vi "Autonomous Independent.vi"   [LabVIEW 2016]
doc: "This VI is called when autonomous begins, and will automatically be terminated when autonomous ends. You can carry out timed or sensor driven robot movement independently without needing to return to the caller."
uses:
  <vilib>/Rock Robotics/WPI/Utilities/WPI_GetSetVariantRefNum.vi
  <vilib>/Rock Robotics/Network Tables/NT Read String.vi
  <vilib>/Rock Robotics/WPI/RobotDrive/WPI_RobotDriveArcadeDrive_Standard(NoSaturation).vi
  <vilib>/Rock Robotics/Network Tables/NT Write Numeric Array.vi
  <vilib>/Rock Robotics/Network Tables/NT Write Boolean.vi
panel:
  # "Be sure to right-click and choose Data Operations>>Make Current Value default if you want to save the array values with the VI"
types:
  T1 = typedef "WPI_JoystickDevRef.ctl" = cluster{"Device":T2}
  T2 = typedef "WPI_JoystickDeviceEnum.ctl" = enum16{"USB 0", "USB 1", "USB 2", "USB 3", "USB 4", "USB 5"}
  T3 = typedef "WPI_RobotDriveDevRef.ctl" = cluster{"DevStatus":errorcluster, "Motors[]":T4[], "Square Inputs":bool, "Max Output":dbl}
  T4 = typedef "WPI_MotorControlDeviceRef.ctl" = cluster{"DeviceStatus":errorcluster, "Type":T5, "PWM":cluster{"PWM Channel":T6, "DeadBand":T7}, "CAN":cluster{"Device Number":u8, "SetOutput VI Ref":variant, "GetOutput VI Ref":variant, "Enable VI Ref":variant, "Disable VI Ref":variant, "Data":variant}, "Invert":bool}
  T5 = typedef "WPI_MotorControlType.ctl" = enum16{"PWM", "CAN"}
  T6 = typedef "FPGA_DIOPWMChannel.ctl" = enum8{"PWM 0", "PWM 1", "PWM 2", "PWM 3", "PWM 4", "PWM 5", "PWM 6", "PWM 7", "PWM 8", "PWM 9", "PWM MXP 0", "PWM MXP 1", "PWM MXP 2", "PWM MXP 3", "PWM MXP 4", "PWM MXP 5", "PWM MXP 6", "PWM MXP 7", "PWM MXP 8", "PWM MXP 9", "Invalid"}
  T7 = typedef "WPI_PWMDeadband.ctl" = cluster{"Name":string, "maxPositivePwm":i32, "minPositivePwm":i32, "centerPwm":i32, "maxNegativePwm":i32, "minNegativePwm":i32, "angularRange":u16}
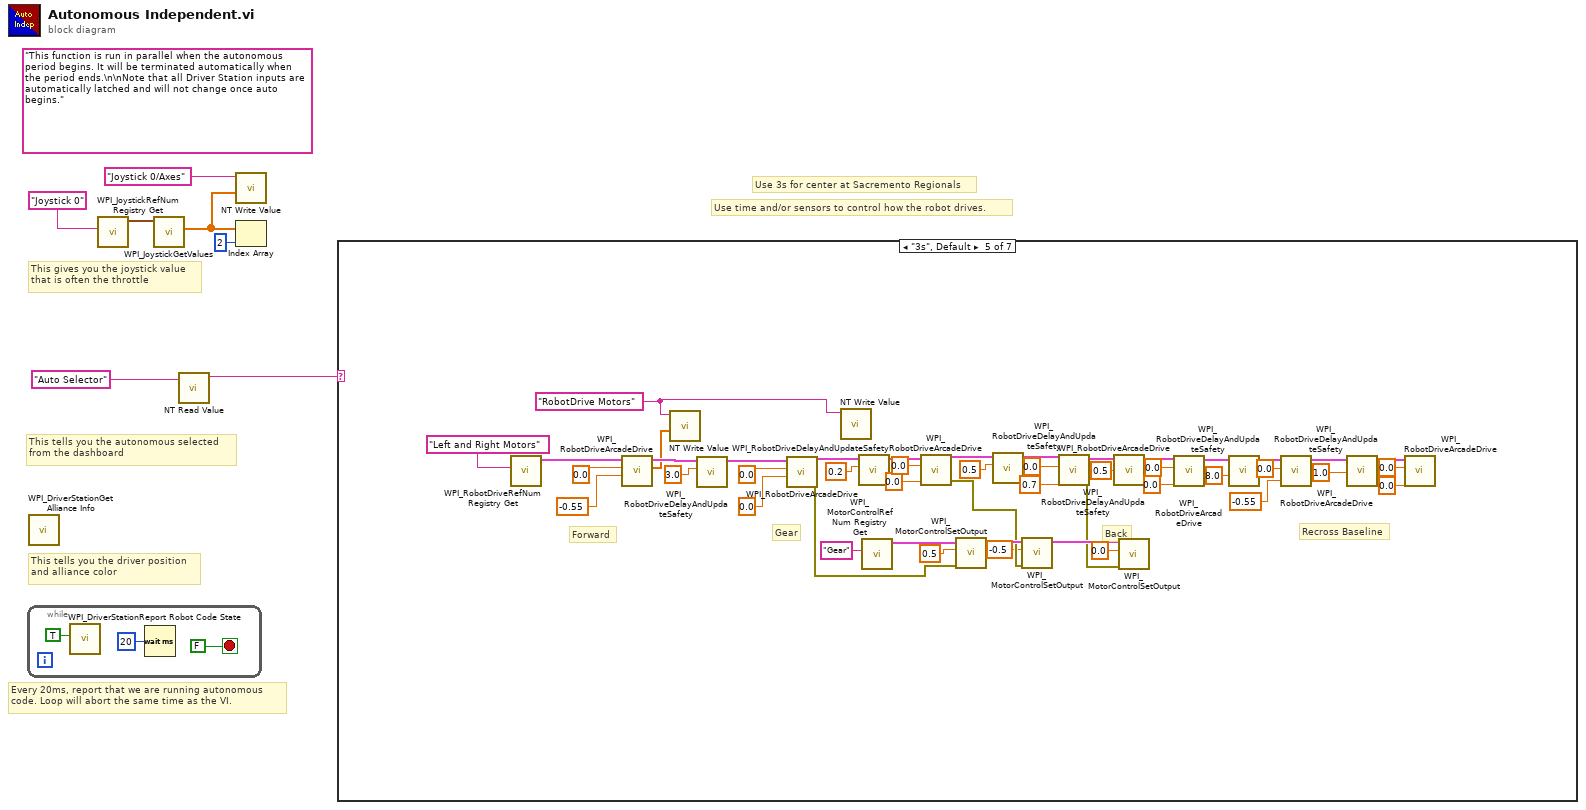
[diagram p0: block diagram]
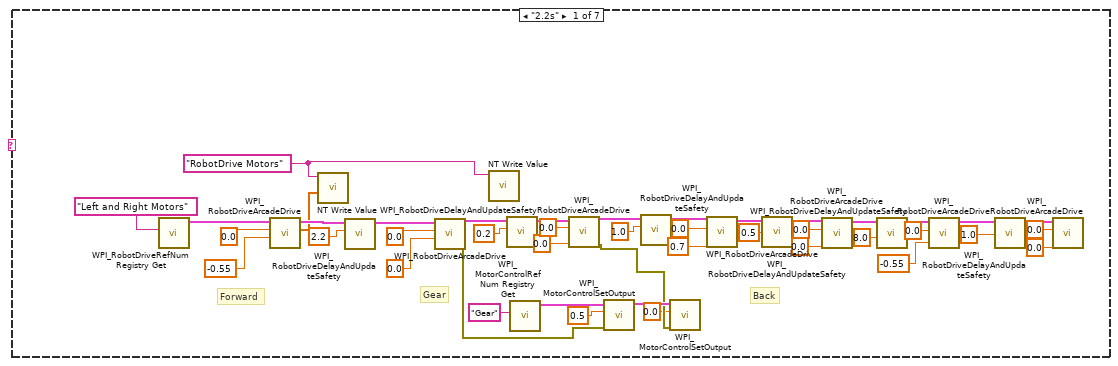
[diagram p2: hidden frame]
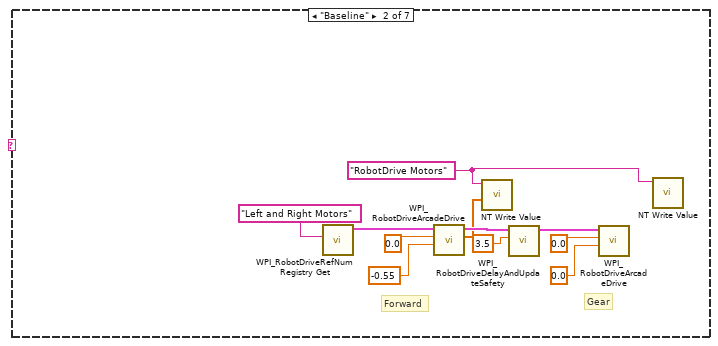
[diagram p3: hidden frame]
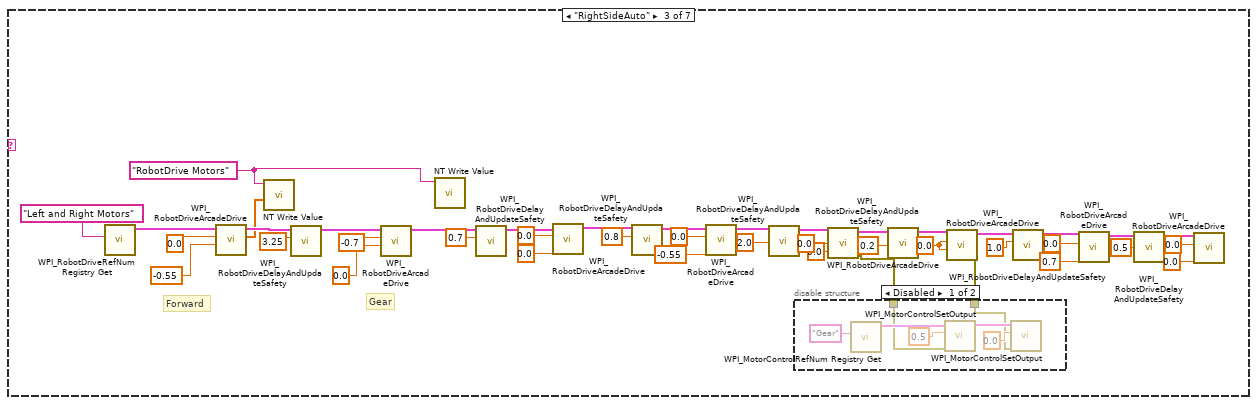
[diagram p4: hidden frame]
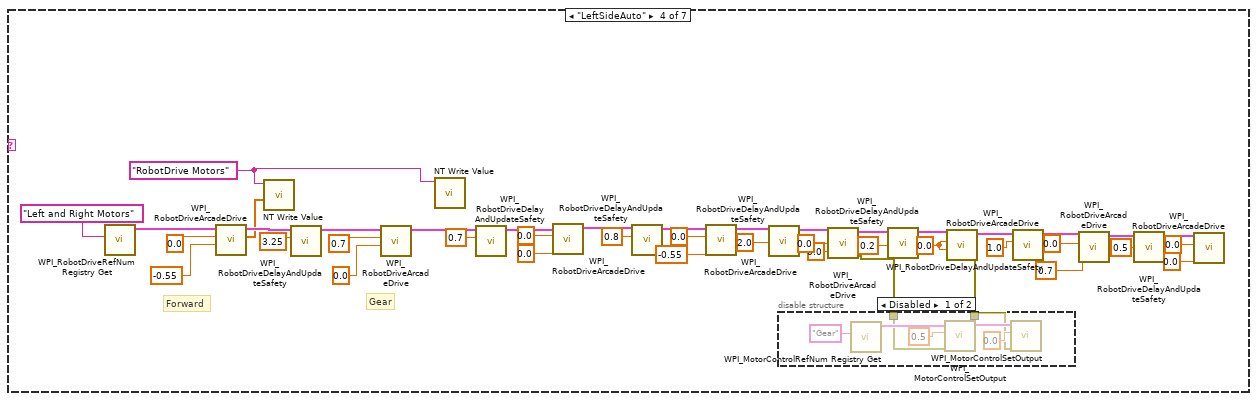
[diagram p6: hidden frame]
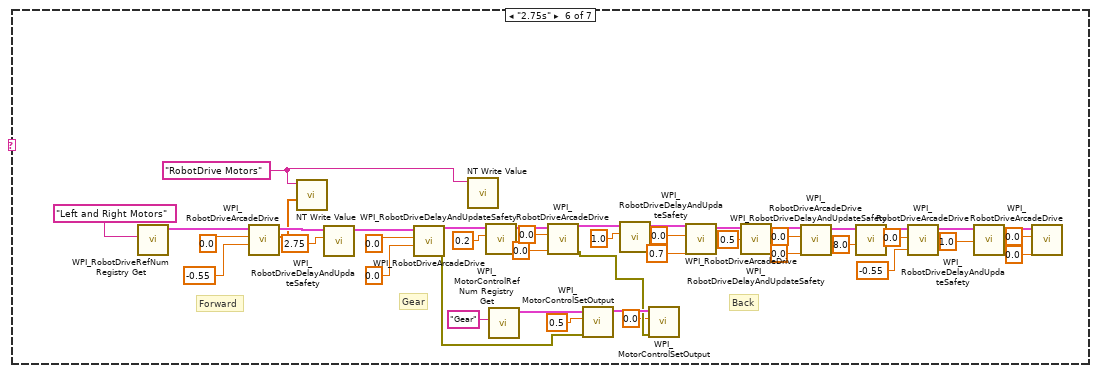
[diagram p8: hidden frame]
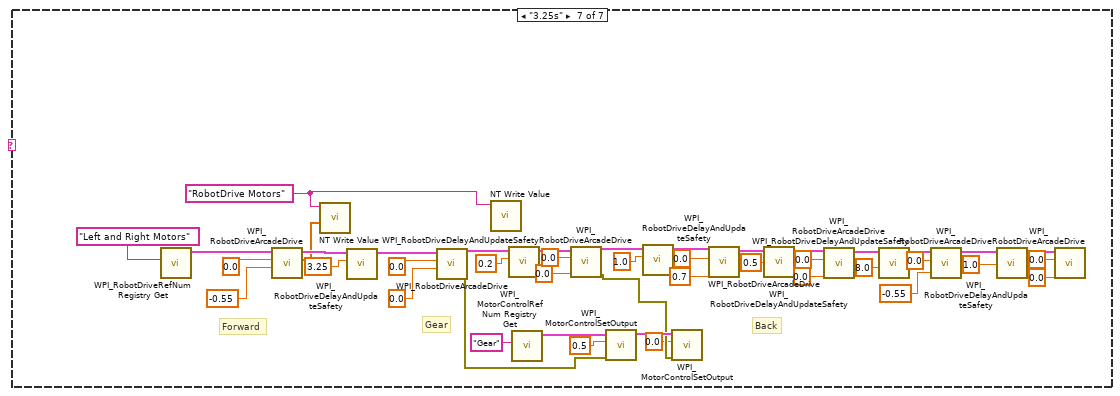
[diagram p9: hidden frame]
diagram:
  (unwired) "This function is run in parallel when the autonomous period begins. It will be terminated automatically when the period ends.\n\nNote that all Driver Station inputs are automatically latched and will not change once auto begins."
  # "Use 3s for center at Sacremento Regionals"
  # "This tells you the autonomous selected\nfrom the dashboard"
  # "Every 20ms, report that we are running autonomous\ncode. Loop will abort the same time as the VI."
  # "This gives you the joystick value\nthat is often the throttle"
  # "Use time and/or sensors to control how the robot drives."
  # "This tells you the driver position\nand alliance color"
  n1 = while {
    stop <- FALSE stop-if-true
    n2 = call <vilib>:"WPI_DriverStationReport Robot Code State.vi"("Autonomous"=TRUE) -> ()  [unwired: 10 in, 1 out]
    n3 = Wait (ms)(milliseconds to wait=u32 20) -> ()  [unwired: 1 out]
  }
  n4 = call <vilib>:"WPI_DriverStationGet Alliance Info.vi"() -> ()  [unwired: 12 out]
  n5 = call <vilib>:"WPI_JoystickRefNum Registry Get.vi"("refnum name"="Joystick 0") -> ("JoystickDevRef"=w6:T1)  [unwired: 1 in, 9 out]
  n6 = call <vilib>:"WPI_JoystickGetValues.vi"("JoystickDevRef"=w6) -> ("Axes"=w2:dbl[])  [unwired: 6 in, 4 out]
  n7 = call-poly <vilib>:"NT Read Value.vi"("Name"="Auto Selector") -> ("String"=w3:string)  [unwired: 9 in, 1 out]
  n8 = call-poly <vilib>:"NT Write Value.vi"("Numeric Array"=w2, "Name"="Joystick 0/Axes") -> ()  [unwired: 9 in, 1 out]
  n9 = Index Array(array=w2, index=2) -> ()  [unwired: 1 out]
  n10 = case shown="\"3s\", Default" w3 {
    frame "2.2s" {
      w47 = "RobotDrive Motors" ("Name")
      # "Back"
      # "Gear"
      # "Forward"
      n11 = call <vilib>:"WPI_RobotDriveRefNum Registry Get.vi"("refnum name"="Left and Right Motors") -> ("RobotDriveDevRef"=w35:T3)  [unwired: 1 in, 9 out]
      n12 = call-poly <vilib>:"WPI_RobotDriveArcadeDrive.vi"("Y axis value"=-0.55 ("X axis value"), "X axis value"=0.0, "RobotDriveDevRef"=w35) -> ("Motor Values"=w46:dbl[], "RobotDriveDevRef"=w52:T3)  [unwired: 1 in, 6 out]
      n13 = call-poly <vilib>:"NT Write Value.vi"("Numeric Array"=w46, "Name"=w47) -> ()  [unwired: 9 in, 1 out]
      n14 = call <vilib>:"WPI_RobotDriveDelayAndUpdateSafety.vi"("Delay (s)"=2.2, "RobotDriveDevRef"=w52) -> ("RobotDriveDevRef 2"=w45:T3)  [unwired: 8 in, 1 out]
      n15 = call-poly <vilib>:"WPI_RobotDriveArcadeDrive.vi"("Y axis value"=0.0 ("X axis value"), "X axis value"=0.0, "RobotDriveDevRef"=w45) -> ("error out"=w25:errorcluster, "RobotDriveDevRef"=w44:T3)  [unwired: 1 in, 6 out]
      n16 = call-poly <vilib>:"NT Write Value.vi"("Name"=w47) -> ()  [unwired: 10 in, 1 out]
      n17 = call <vilib>:"WPI_RobotDriveDelayAndUpdateSafety.vi"("Delay (s)"=0.2, "RobotDriveDevRef"=w44) -> ("RobotDriveDevRef 2"=w29:T3)  [unwired: 8 in, 1 out]
      n18 = call <vilib>:"WPI_MotorControlRefNum Registry Get.vi"("refnum name"="Gear") -> ("MotorControlDevRef"=w33:T4)  [unwired: 9 in, 1 out]
      n19 = call-poly <vilib>:"WPI_RobotDriveArcadeDrive.vi"("Y axis value"=0.0, "X axis value"=0.0, "RobotDriveDevRef"=w29) -> ("error out"=w23:errorcluster, "RobotDriveDevRef"=w30:T3)  [unwired: 1 in, 6 out]
      n20 = call <vilib>:"WPI_MotorControlSetOutput.vi"("error in (no error)"=w25, "Output"=0.5, "MotorControlDevRef"=w33) -> ("MotorControlDevRef"=w24:T4)  [unwired: 6 in, 2 out]
      n21 = call <vilib>:"WPI_RobotDriveDelayAndUpdateSafety.vi"("Delay (s)"=1.0, "RobotDriveDevRef"=w30) -> ("RobotDriveDevRef 2"=w28:T3)  [unwired: 8 in, 1 out]
      n22 = call <vilib>:"WPI_MotorControlSetOutput.vi"("error in (no error)"=w23, "Output"=0.0, "MotorControlDevRef"=w24) -> ()  [unwired: 6 in, 3 out]
      n23 = call-poly <vilib>:"WPI_RobotDriveArcadeDrive.vi"("Y axis value"=0.7, "X axis value"=0.0, "RobotDriveDevRef"=w28) -> ("RobotDriveDevRef"=w40:T3)  [unwired: 1 in, 7 out]
      n24 = call <vilib>:"WPI_RobotDriveDelayAndUpdateSafety.vi"("Delay (s)"=0.5, "RobotDriveDevRef"=w40) -> ("RobotDriveDevRef 2"=w38:T3)  [unwired: 8 in, 1 out]
      n25 = call-poly <vilib>:"WPI_RobotDriveArcadeDrive.vi"("Y axis value"=0.0, "X axis value"=0.0, "RobotDriveDevRef"=w38) -> ("RobotDriveDevRef"=w21:T3)  [unwired: 1 in, 7 out]
      n26 = call <vilib>:"WPI_RobotDriveDelayAndUpdateSafety.vi"("Delay (s)"=8.0, "RobotDriveDevRef"=w21) -> ("RobotDriveDevRef 2"=w19:T3)  [unwired: 8 in, 1 out]
      n27 = call-poly <vilib>:"WPI_RobotDriveArcadeDrive.vi"("Y axis value"=-0.55, "X axis value"=0.0, "RobotDriveDevRef"=w19) -> ("RobotDriveDevRef"=w16:T3)  [unwired: 1 in, 7 out]
      n28 = call <vilib>:"WPI_RobotDriveDelayAndUpdateSafety.vi"("Delay (s)"=1.0, "RobotDriveDevRef"=w16) -> ("RobotDriveDevRef 2"=w14:T3)  [unwired: 8 in, 1 out]
      n29 = call-poly <vilib>:"WPI_RobotDriveArcadeDrive.vi"("Y axis value"=0.0, "X axis value"=0.0, "RobotDriveDevRef"=w14) -> ()  [unwired: 1 in, 8 out]
    }
    frame "Baseline" {
      w55 = "RobotDrive Motors" ("Name")
      # "Gear"
      # "Forward"
      n30 = call <vilib>:"WPI_RobotDriveRefNum Registry Get.vi"("refnum name"="Left and Right Motors") -> ("RobotDriveDevRef"=w56:T3)  [unwired: 1 in, 9 out]
      n31 = call-poly <vilib>:"WPI_RobotDriveArcadeDrive.vi"("Y axis value"=-0.55 ("X axis value"), "X axis value"=0.0, "RobotDriveDevRef"=w56) -> ("Motor Values"=w58:dbl[], "RobotDriveDevRef"=w63:T3)  [unwired: 1 in, 6 out]
      n32 = call-poly <vilib>:"NT Write Value.vi"("Numeric Array"=w58, "Name"=w55) -> ()  [unwired: 9 in, 1 out]
      n33 = call <vilib>:"WPI_RobotDriveDelayAndUpdateSafety.vi"("Delay (s)"=3.5, "RobotDriveDevRef"=w63) -> ("RobotDriveDevRef 2"=w57:T3)  [unwired: 8 in, 1 out]
      n34 = call-poly <vilib>:"WPI_RobotDriveArcadeDrive.vi"("Y axis value"=0.0 ("X axis value"), "X axis value"=0.0, "RobotDriveDevRef"=w57) -> ()  [unwired: 1 in, 8 out]
      n35 = call-poly <vilib>:"NT Write Value.vi"("Name"=w55) -> ()  [unwired: 10 in, 1 out]
    }
    frame "RightSideAuto" {
      w67 = 0.0 ("X axis value")
      w97 = "RobotDrive Motors" ("Name")
      # "Gear"
      # "Forward"
      n36 = call <vilib>:"WPI_RobotDriveRefNum Registry Get.vi"("refnum name"="Left and Right Motors") -> ("RobotDriveDevRef"=w98:T3)  [unwired: 1 in, 9 out]
      n37 = call-poly <vilib>:"WPI_RobotDriveArcadeDrive.vi"("Y axis value"=-0.55 ("X axis value"), "X axis value"=0.0, "RobotDriveDevRef"=w98) -> ("Motor Values"=w100:dbl[], "RobotDriveDevRef"=w105:T3)  [unwired: 1 in, 6 out]
      n38 = call-poly <vilib>:"NT Write Value.vi"("Numeric Array"=w100, "Name"=w97) -> ()  [unwired: 9 in, 1 out]
      n39 = call <vilib>:"WPI_RobotDriveDelayAndUpdateSafety.vi"("Delay (s)"=3.25, "RobotDriveDevRef"=w105) -> ("RobotDriveDevRef 2"=w99:T3)  [unwired: 8 in, 1 out]
      n40 = call-poly <vilib>:"WPI_RobotDriveArcadeDrive.vi"("Y axis value"=0.0 ("X axis value"), "X axis value"=-0.7, "RobotDriveDevRef"=w99) -> ("RobotDriveDevRef"=w95:T3)  [unwired: 1 in, 7 out]
      n41 = call-poly <vilib>:"NT Write Value.vi"("Name"=w97) -> ()  [unwired: 10 in, 1 out]
      n42 = call <vilib>:"WPI_RobotDriveDelayAndUpdateSafety.vi"("Delay (s)"=0.7, "RobotDriveDevRef"=w95) -> ("RobotDriveDevRef 2"=w93:T3)  [unwired: 8 in, 1 out]
      n43 = call-poly <vilib>:"WPI_RobotDriveArcadeDrive.vi"("Y axis value"=0.0, "X axis value"=0.0, "RobotDriveDevRef"=w93) -> ("RobotDriveDevRef"=w90:T3)  [unwired: 1 in, 7 out]
      n44 = call <vilib>:"WPI_RobotDriveDelayAndUpdateSafety.vi"("Delay (s)"=0.8, "RobotDriveDevRef"=w90) -> ("RobotDriveDevRef 2"=w88:T3)  [unwired: 8 in, 1 out]
      n45 = call-poly <vilib>:"WPI_RobotDriveArcadeDrive.vi"("Y axis value"=-0.55, "X axis value"=0.0, "RobotDriveDevRef"=w88) -> ("RobotDriveDevRef"=w85:T3)  [unwired: 1 in, 7 out]
      n46 = call <vilib>:"WPI_RobotDriveDelayAndUpdateSafety.vi"("Delay (s)"=2.0, "RobotDriveDevRef"=w85) -> ("RobotDriveDevRef 2"=w81:T3)  [unwired: 8 in, 1 out]
      n47 = call-poly <vilib>:"WPI_RobotDriveArcadeDrive.vi"("Y axis value"=0.0, "X axis value"=0.0, "RobotDriveDevRef"=w81) -> ("error out"=w72:errorcluster, "RobotDriveDevRef"=w70:T3)  [unwired: 1 in, 6 out]
      n48 = call <vilib>:"WPI_RobotDriveDelayAndUpdateSafety.vi"("Delay (s)"=0.2, "RobotDriveDevRef"=w70) -> ("RobotDriveDevRef 2"=w71:T3)  [unwired: 8 in, 1 out]
      n49 = call-poly <vilib>:"WPI_RobotDriveArcadeDrive.vi"("Y axis value"=w67, "X axis value"=w67, "RobotDriveDevRef"=w71) -> ("error out"=w68:errorcluster, "RobotDriveDevRef"=w65:T3)  [unwired: 1 in, 6 out]
      n50 = disable-structure shown="Disabled" {
        disable-tunnel: w72 -> [w108 _]
        disable-tunnel: w68 -> [w107 _]
        frame Disabled {
          n51 = call <vilib>:"WPI_MotorControlRefNum Registry Get.vi"("refnum name"="Gear") -> ("MotorControlDevRef"=w112:T4)  [unwired: 9 in, 1 out]
          n52 = call <vilib>:"WPI_MotorControlSetOutput.vi"("error in (no error)"=w108, "Output"=0.5, "MotorControlDevRef"=w112) -> ("MotorControlDevRef"=w109:T4)  [unwired: 6 in, 2 out]
          n53 = call <vilib>:"WPI_MotorControlSetOutput.vi"("error in (no error)"=w107, "Output"=0.0, "MotorControlDevRef"=w109) -> ()  [unwired: 6 in, 3 out]
        }
        frame Enabled {
        }
      }
      n54 = call <vilib>:"WPI_RobotDriveDelayAndUpdateSafety.vi"("Delay (s)"=1.0, "RobotDriveDevRef"=w65) -> ("RobotDriveDevRef 2"=w73:T3)  [unwired: 8 in, 1 out]
      n55 = call-poly <vilib>:"WPI_RobotDriveArcadeDrive.vi"("Y axis value"=0.7, "X axis value"=0.0, "RobotDriveDevRef"=w73) -> ("RobotDriveDevRef"=w78:T3)  [unwired: 1 in, 7 out]
      n56 = call <vilib>:"WPI_RobotDriveDelayAndUpdateSafety.vi"("Delay (s)"=0.5, "RobotDriveDevRef"=w78) -> ("RobotDriveDevRef 2"=w76:T3)  [unwired: 8 in, 1 out]
      n57 = call-poly <vilib>:"WPI_RobotDriveArcadeDrive.vi"("Y axis value"=0.0, "X axis value"=0.0, "RobotDriveDevRef"=w76) -> ()  [unwired: 1 in, 8 out]
    }
    frame "LeftSideAuto" {
      w116 = 0.0 ("X axis value")
      w146 = "RobotDrive Motors" ("Name")
      # "Gear"
      # "Forward"
      n58 = call <vilib>:"WPI_RobotDriveRefNum Registry Get.vi"("refnum name"="Left and Right Motors") -> ("RobotDriveDevRef"=w147:T3)  [unwired: 1 in, 9 out]
      n59 = call-poly <vilib>:"WPI_RobotDriveArcadeDrive.vi"("Y axis value"=-0.55 ("X axis value"), "X axis value"=0.0, "RobotDriveDevRef"=w147) -> ("Motor Values"=w149:dbl[], "RobotDriveDevRef"=w154:T3)  [unwired: 1 in, 6 out]
      n60 = call-poly <vilib>:"NT Write Value.vi"("Numeric Array"=w149, "Name"=w146) -> ()  [unwired: 9 in, 1 out]
      n61 = call <vilib>:"WPI_RobotDriveDelayAndUpdateSafety.vi"("Delay (s)"=3.25, "RobotDriveDevRef"=w154) -> ("RobotDriveDevRef 2"=w148:T3)  [unwired: 8 in, 1 out]
      n62 = call-poly <vilib>:"WPI_RobotDriveArcadeDrive.vi"("Y axis value"=0.0 ("X axis value"), "X axis value"=0.7, "RobotDriveDevRef"=w148) -> ("RobotDriveDevRef"=w144:T3)  [unwired: 1 in, 7 out]
      n63 = call-poly <vilib>:"NT Write Value.vi"("Name"=w146) -> ()  [unwired: 10 in, 1 out]
      n64 = call <vilib>:"WPI_RobotDriveDelayAndUpdateSafety.vi"("Delay (s)"=0.7, "RobotDriveDevRef"=w144) -> ("RobotDriveDevRef 2"=w142:T3)  [unwired: 8 in, 1 out]
      n65 = call-poly <vilib>:"WPI_RobotDriveArcadeDrive.vi"("Y axis value"=0.0, "X axis value"=0.0, "RobotDriveDevRef"=w142) -> ("RobotDriveDevRef"=w139:T3)  [unwired: 1 in, 7 out]
      n66 = call <vilib>:"WPI_RobotDriveDelayAndUpdateSafety.vi"("Delay (s)"=0.8, "RobotDriveDevRef"=w139) -> ("RobotDriveDevRef 2"=w137:T3)  [unwired: 8 in, 1 out]
      n67 = call-poly <vilib>:"WPI_RobotDriveArcadeDrive.vi"("Y axis value"=-0.55, "X axis value"=0.0, "RobotDriveDevRef"=w137) -> ("RobotDriveDevRef"=w134:T3)  [unwired: 1 in, 7 out]
      n68 = call <vilib>:"WPI_RobotDriveDelayAndUpdateSafety.vi"("Delay (s)"=2.0, "RobotDriveDevRef"=w134) -> ("RobotDriveDevRef 2"=w130:T3)  [unwired: 8 in, 1 out]
      n69 = call-poly <vilib>:"WPI_RobotDriveArcadeDrive.vi"("Y axis value"=0.0, "X axis value"=0.0, "RobotDriveDevRef"=w130) -> ("error out"=w121:errorcluster, "RobotDriveDevRef"=w119:T3)  [unwired: 1 in, 6 out]
      n70 = call <vilib>:"WPI_RobotDriveDelayAndUpdateSafety.vi"("Delay (s)"=0.2, "RobotDriveDevRef"=w119) -> ("RobotDriveDevRef 2"=w120:T3)  [unwired: 8 in, 1 out]
      n71 = call-poly <vilib>:"WPI_RobotDriveArcadeDrive.vi"("Y axis value"=w116, "X axis value"=w116, "RobotDriveDevRef"=w120) -> ("error out"=w117:errorcluster, "RobotDriveDevRef"=w114:T3)  [unwired: 1 in, 6 out]
      n72 = disable-structure shown="Disabled" {
        disable-tunnel: w121 -> [w157 _]
        disable-tunnel: w117 -> [w156 _]
        frame Disabled {
          n73 = call <vilib>:"WPI_MotorControlRefNum Registry Get.vi"("refnum name"="Gear") -> ("MotorControlDevRef"=w161:T4)  [unwired: 9 in, 1 out]
          n74 = call <vilib>:"WPI_MotorControlSetOutput.vi"("error in (no error)"=w157, "Output"=0.5, "MotorControlDevRef"=w161) -> ("MotorControlDevRef"=w158:T4)  [unwired: 6 in, 2 out]
          n75 = call <vilib>:"WPI_MotorControlSetOutput.vi"("error in (no error)"=w156, "Output"=0.0, "MotorControlDevRef"=w158) -> ()  [unwired: 6 in, 3 out]
        }
        frame Enabled {
        }
      }
      n76 = call <vilib>:"WPI_RobotDriveDelayAndUpdateSafety.vi"("Delay (s)"=1.0, "RobotDriveDevRef"=w114) -> ("RobotDriveDevRef 2"=w122:T3)  [unwired: 8 in, 1 out]
      n77 = call-poly <vilib>:"WPI_RobotDriveArcadeDrive.vi"("Y axis value"=0.7, "X axis value"=0.0, "RobotDriveDevRef"=w122) -> ("RobotDriveDevRef"=w127:T3)  [unwired: 1 in, 7 out]
      n78 = call <vilib>:"WPI_RobotDriveDelayAndUpdateSafety.vi"("Delay (s)"=0.5, "RobotDriveDevRef"=w127) -> ("RobotDriveDevRef 2"=w125:T3)  [unwired: 8 in, 1 out]
      n79 = call-poly <vilib>:"WPI_RobotDriveArcadeDrive.vi"("Y axis value"=0.0, "X axis value"=0.0, "RobotDriveDevRef"=w125) -> ()  [unwired: 1 in, 8 out]
    }
    frame "3s", Default {
      w201 = "RobotDrive Motors" ("Name")
      # "Recross Baseline"
      # "Back"
      # "Gear"
      # "Forward"
      n80 = call <vilib>:"WPI_RobotDriveRefNum Registry Get.vi"("refnum name"="Left and Right Motors") -> ("RobotDriveDevRef"=w189:T3)  [unwired: 1 in, 9 out]
      n81 = call-poly <vilib>:"WPI_RobotDriveArcadeDrive.vi"("Y axis value"=-0.55 ("X axis value"), "X axis value"=0.0, "RobotDriveDevRef"=w189) -> ("Motor Values"=w200:dbl[], "RobotDriveDevRef"=w206:T3)  [unwired: 1 in, 6 out]
      n82 = call-poly <vilib>:"NT Write Value.vi"("Numeric Array"=w200, "Name"=w201) -> ()  [unwired: 9 in, 1 out]
      n83 = call <vilib>:"WPI_RobotDriveDelayAndUpdateSafety.vi"("Delay (s)"=3.0, "RobotDriveDevRef"=w206) -> ("RobotDriveDevRef 2"=w199:T3)  [unwired: 8 in, 1 out]
      n84 = call-poly <vilib>:"WPI_RobotDriveArcadeDrive.vi"("Y axis value"=0.0 ("X axis value"), "X axis value"=0.0, "RobotDriveDevRef"=w199) -> ("error out"=w179:errorcluster, "RobotDriveDevRef"=w198:T3)  [unwired: 1 in, 6 out]
      n85 = call-poly <vilib>:"NT Write Value.vi"("Name"=w201) -> ()  [unwired: 10 in, 1 out]
      n86 = call <vilib>:"WPI_RobotDriveDelayAndUpdateSafety.vi"("Delay (s)"=0.2, "RobotDriveDevRef"=w198) -> ("RobotDriveDevRef 2"=w183:T3)  [unwired: 8 in, 1 out]
      n87 = call <vilib>:"WPI_MotorControlRefNum Registry Get.vi"("refnum name"="Gear") -> ("MotorControlDevRef"=w187:T4)  [unwired: 9 in, 1 out]
      n88 = call-poly <vilib>:"WPI_RobotDriveArcadeDrive.vi"("Y axis value"=0.0, "X axis value"=0.0, "RobotDriveDevRef"=w183) -> ("error out"=w177:errorcluster, "RobotDriveDevRef"=w184:T3)  [unwired: 1 in, 6 out]
      n89 = call <vilib>:"WPI_MotorControlSetOutput.vi"("error in (no error)"=w179, "Output"=0.5, "MotorControlDevRef"=w187) -> ("MotorControlDevRef"=w178:T4)  [unwired: 6 in, 2 out]
      n90 = call <vilib>:"WPI_RobotDriveDelayAndUpdateSafety.vi"("Delay (s)"=0.5, "RobotDriveDevRef"=w184) -> ("RobotDriveDevRef 2"=w182:T3)  [unwired: 8 in, 1 out]
      n91 = call <vilib>:"WPI_MotorControlSetOutput.vi"("error in (no error)"=w177, "Output"=-0.5, "MotorControlDevRef"=w178) -> ("MotorControlDevRef"=w165:T4)  [unwired: 6 in, 2 out]
      n92 = call-poly <vilib>:"WPI_RobotDriveArcadeDrive.vi"("Y axis value"=0.7, "X axis value"=0.0, "RobotDriveDevRef"=w182) -> ("error out"=w163:errorcluster, "RobotDriveDevRef"=w194:T3)  [unwired: 1 in, 6 out]
      n93 = call <vilib>:"WPI_RobotDriveDelayAndUpdateSafety.vi"("Delay (s)"=0.5, "RobotDriveDevRef"=w194) -> ("RobotDriveDevRef 2"=w192:T3)  [unwired: 8 in, 1 out]
      n94 = call <vilib>:"WPI_MotorControlSetOutput.vi"("error in (no error)"=w163, "Output"=0.0, "MotorControlDevRef"=w165) -> ()  [unwired: 6 in, 3 out]
      n95 = call-poly <vilib>:"WPI_RobotDriveArcadeDrive.vi"("Y axis value"=0.0, "X axis value"=0.0, "RobotDriveDevRef"=w192) -> ("RobotDriveDevRef"=w175:T3)  [unwired: 1 in, 7 out]
      n96 = call <vilib>:"WPI_RobotDriveDelayAndUpdateSafety.vi"("Delay (s)"=8.0, "RobotDriveDevRef"=w175) -> ("RobotDriveDevRef 2"=w173:T3)  [unwired: 8 in, 1 out]
      n97 = call-poly <vilib>:"WPI_RobotDriveArcadeDrive.vi"("Y axis value"=-0.55, "X axis value"=0.0, "RobotDriveDevRef"=w173) -> ("RobotDriveDevRef"=w170:T3)  [unwired: 1 in, 7 out]
      n98 = call <vilib>:"WPI_RobotDriveDelayAndUpdateSafety.vi"("Delay (s)"=1.0, "RobotDriveDevRef"=w170) -> ("RobotDriveDevRef 2"=w168:T3)  [unwired: 8 in, 1 out]
      n99 = call-poly <vilib>:"WPI_RobotDriveArcadeDrive.vi"("Y axis value"=0.0, "X axis value"=0.0, "RobotDriveDevRef"=w168) -> ()  [unwired: 1 in, 8 out]
    }
    frame "2.75s" {
      w244 = "RobotDrive Motors" ("Name")
      # "Back"
      # "Gear"
      # "Forward"
      n100 = call <vilib>:"WPI_RobotDriveRefNum Registry Get.vi"("refnum name"="Left and Right Motors") -> ("RobotDriveDevRef"=w232:T3)  [unwired: 1 in, 9 out]
      n101 = call-poly <vilib>:"WPI_RobotDriveArcadeDrive.vi"("Y axis value"=-0.55 ("X axis value"), "X axis value"=0.0, "RobotDriveDevRef"=w232) -> ("Motor Values"=w243:dbl[], "RobotDriveDevRef"=w249:T3)  [unwired: 1 in, 6 out]
      n102 = call-poly <vilib>:"NT Write Value.vi"("Numeric Array"=w243, "Name"=w244) -> ()  [unwired: 9 in, 1 out]
      n103 = call <vilib>:"WPI_RobotDriveDelayAndUpdateSafety.vi"("Delay (s)"=2.75, "RobotDriveDevRef"=w249) -> ("RobotDriveDevRef 2"=w242:T3)  [unwired: 8 in, 1 out]
      n104 = call-poly <vilib>:"WPI_RobotDriveArcadeDrive.vi"("Y axis value"=0.0 ("X axis value"), "X axis value"=0.0, "RobotDriveDevRef"=w242) -> ("error out"=w222:errorcluster, "RobotDriveDevRef"=w241:T3)  [unwired: 1 in, 6 out]
      n105 = call-poly <vilib>:"NT Write Value.vi"("Name"=w244) -> ()  [unwired: 10 in, 1 out]
      n106 = call <vilib>:"WPI_RobotDriveDelayAndUpdateSafety.vi"("Delay (s)"=0.2, "RobotDriveDevRef"=w241) -> ("RobotDriveDevRef 2"=w226:T3)  [unwired: 8 in, 1 out]
      n107 = call <vilib>:"WPI_MotorControlRefNum Registry Get.vi"("refnum name"="Gear") -> ("MotorControlDevRef"=w230:T4)  [unwired: 9 in, 1 out]
      n108 = call-poly <vilib>:"WPI_RobotDriveArcadeDrive.vi"("Y axis value"=0.0, "X axis value"=0.0, "RobotDriveDevRef"=w226) -> ("error out"=w220:errorcluster, "RobotDriveDevRef"=w227:T3)  [unwired: 1 in, 6 out]
      n109 = call <vilib>:"WPI_MotorControlSetOutput.vi"("error in (no error)"=w222, "Output"=0.5, "MotorControlDevRef"=w230) -> ("MotorControlDevRef"=w221:T4)  [unwired: 6 in, 2 out]
      n110 = call <vilib>:"WPI_RobotDriveDelayAndUpdateSafety.vi"("Delay (s)"=1.0, "RobotDriveDevRef"=w227) -> ("RobotDriveDevRef 2"=w225:T3)  [unwired: 8 in, 1 out]
      n111 = call <vilib>:"WPI_MotorControlSetOutput.vi"("error in (no error)"=w220, "Output"=0.0, "MotorControlDevRef"=w221) -> ()  [unwired: 6 in, 3 out]
      n112 = call-poly <vilib>:"WPI_RobotDriveArcadeDrive.vi"("Y axis value"=0.7, "X axis value"=0.0, "RobotDriveDevRef"=w225) -> ("RobotDriveDevRef"=w237:T3)  [unwired: 1 in, 7 out]
      n113 = call <vilib>:"WPI_RobotDriveDelayAndUpdateSafety.vi"("Delay (s)"=0.5, "RobotDriveDevRef"=w237) -> ("RobotDriveDevRef 2"=w235:T3)  [unwired: 8 in, 1 out]
      n114 = call-poly <vilib>:"WPI_RobotDriveArcadeDrive.vi"("Y axis value"=0.0, "X axis value"=0.0, "RobotDriveDevRef"=w235) -> ("RobotDriveDevRef"=w218:T3)  [unwired: 1 in, 7 out]
      n115 = call <vilib>:"WPI_RobotDriveDelayAndUpdateSafety.vi"("Delay (s)"=8.0, "RobotDriveDevRef"=w218) -> ("RobotDriveDevRef 2"=w216:T3)  [unwired: 8 in, 1 out]
      n116 = call-poly <vilib>:"WPI_RobotDriveArcadeDrive.vi"("Y axis value"=-0.55, "X axis value"=0.0, "RobotDriveDevRef"=w216) -> ("RobotDriveDevRef"=w213:T3)  [unwired: 1 in, 7 out]
      n117 = call <vilib>:"WPI_RobotDriveDelayAndUpdateSafety.vi"("Delay (s)"=1.0, "RobotDriveDevRef"=w213) -> ("RobotDriveDevRef 2"=w211:T3)  [unwired: 8 in, 1 out]
      n118 = call-poly <vilib>:"WPI_RobotDriveArcadeDrive.vi"("Y axis value"=0.0, "X axis value"=0.0, "RobotDriveDevRef"=w211) -> ()  [unwired: 1 in, 8 out]
    }
    frame "3.25s" {
      w287 = "RobotDrive Motors" ("Name")
      # "Back"
      # "Gear"
      # "Forward"
      n119 = call <vilib>:"WPI_RobotDriveRefNum Registry Get.vi"("refnum name"="Left and Right Motors") -> ("RobotDriveDevRef"=w275:T3)  [unwired: 1 in, 9 out]
      n120 = call-poly <vilib>:"WPI_RobotDriveArcadeDrive.vi"("Y axis value"=-0.55 ("X axis value"), "X axis value"=0.0, "RobotDriveDevRef"=w275) -> ("Motor Values"=w286:dbl[], "RobotDriveDevRef"=w292:T3)  [unwired: 1 in, 6 out]
      n121 = call-poly <vilib>:"NT Write Value.vi"("Numeric Array"=w286, "Name"=w287) -> ()  [unwired: 9 in, 1 out]
      n122 = call <vilib>:"WPI_RobotDriveDelayAndUpdateSafety.vi"("Delay (s)"=3.25, "RobotDriveDevRef"=w292) -> ("RobotDriveDevRef 2"=w285:T3)  [unwired: 8 in, 1 out]
      n123 = call-poly <vilib>:"WPI_RobotDriveArcadeDrive.vi"("Y axis value"=0.0 ("X axis value"), "X axis value"=0.0, "RobotDriveDevRef"=w285) -> ("error out"=w265:errorcluster, "RobotDriveDevRef"=w284:T3)  [unwired: 1 in, 6 out]
      n124 = call-poly <vilib>:"NT Write Value.vi"("Name"=w287) -> ()  [unwired: 10 in, 1 out]
      n125 = call <vilib>:"WPI_RobotDriveDelayAndUpdateSafety.vi"("Delay (s)"=0.2, "RobotDriveDevRef"=w284) -> ("RobotDriveDevRef 2"=w269:T3)  [unwired: 8 in, 1 out]
      n126 = call <vilib>:"WPI_MotorControlRefNum Registry Get.vi"("refnum name"="Gear") -> ("MotorControlDevRef"=w273:T4)  [unwired: 9 in, 1 out]
      n127 = call-poly <vilib>:"WPI_RobotDriveArcadeDrive.vi"("Y axis value"=0.0, "X axis value"=0.0, "RobotDriveDevRef"=w269) -> ("error out"=w263:errorcluster, "RobotDriveDevRef"=w270:T3)  [unwired: 1 in, 6 out]
      n128 = call <vilib>:"WPI_MotorControlSetOutput.vi"("error in (no error)"=w265, "Output"=0.5, "MotorControlDevRef"=w273) -> ("MotorControlDevRef"=w264:T4)  [unwired: 6 in, 2 out]
      n129 = call <vilib>:"WPI_RobotDriveDelayAndUpdateSafety.vi"("Delay (s)"=1.0, "RobotDriveDevRef"=w270) -> ("RobotDriveDevRef 2"=w268:T3)  [unwired: 8 in, 1 out]
      n130 = call <vilib>:"WPI_MotorControlSetOutput.vi"("error in (no error)"=w263, "Output"=0.0, "MotorControlDevRef"=w264) -> ()  [unwired: 6 in, 3 out]
      n131 = call-poly <vilib>:"WPI_RobotDriveArcadeDrive.vi"("Y axis value"=0.7, "X axis value"=0.0, "RobotDriveDevRef"=w268) -> ("RobotDriveDevRef"=w280:T3)  [unwired: 1 in, 7 out]
      n132 = call <vilib>:"WPI_RobotDriveDelayAndUpdateSafety.vi"("Delay (s)"=0.5, "RobotDriveDevRef"=w280) -> ("RobotDriveDevRef 2"=w278:T3)  [unwired: 8 in, 1 out]
      n133 = call-poly <vilib>:"WPI_RobotDriveArcadeDrive.vi"("Y axis value"=0.0, "X axis value"=0.0, "RobotDriveDevRef"=w278) -> ("RobotDriveDevRef"=w261:T3)  [unwired: 1 in, 7 out]
      n134 = call <vilib>:"WPI_RobotDriveDelayAndUpdateSafety.vi"("Delay (s)"=8.0, "RobotDriveDevRef"=w261) -> ("RobotDriveDevRef 2"=w259:T3)  [unwired: 8 in, 1 out]
      n135 = call-poly <vilib>:"WPI_RobotDriveArcadeDrive.vi"("Y axis value"=-0.55, "X axis value"=0.0, "RobotDriveDevRef"=w259) -> ("RobotDriveDevRef"=w256:T3)  [unwired: 1 in, 7 out]
      n136 = call <vilib>:"WPI_RobotDriveDelayAndUpdateSafety.vi"("Delay (s)"=1.0, "RobotDriveDevRef"=w256) -> ("RobotDriveDevRef 2"=w254:T3)  [unwired: 8 in, 1 out]
      n137 = call-poly <vilib>:"WPI_RobotDriveArcadeDrive.vi"("Y axis value"=0.0, "X axis value"=0.0, "RobotDriveDevRef"=w254) -> ()  [unwired: 1 in, 8 out]
    }
  }
